vi "Main.vi"   [LabVIEW 2021]
uses:
  Dev Actor/Dev Actor/Dev Actor.lvclass
  C:/git/jettl/src/Actor/Actor/Actor.lvclass
  jettl/jettl/jettl.lvclass
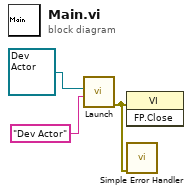
[diagram p0: block diagram]
diagram:
  n1 = call "Launch.vi"("Alias"="Dev Actor", "Actor"=refnum<class "Dev Actor.lvclass"> refnum ("Dev Actor.lvlib:Dev Actor.lvclass")) -> ("error out"=w2:errorcluster)  [unwired: 9 in]
  n2 = invoke class="VI" method="FP.Close"(error in=w2) -> ()  [unwired: 2 in, 3 out]
  n3 = call <vilib>:"Simple Error Handler.vi"("error in (no error)"=w2) -> ()  [unwired: 4 in, 5 out]
